vi "readShopInfo.vi"() -> (0 "数组 2":T1(array[cluster]))   [LabVIEW 2013, in "ShopBase.lvclass"]
uses:
  ShopBase.lvclass
  <vilib>/Utility/xml.llb/Read From XML File(string).vi
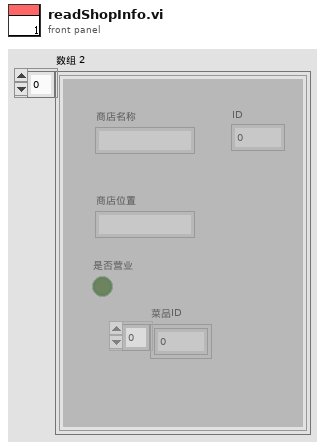
[diagram p1: front panel]
types:
  T1 = cluster{"ID":dbl, "商店名称":string, "商店位置":string, "是否营业":bool, "菜品ID":dbl[]}[]
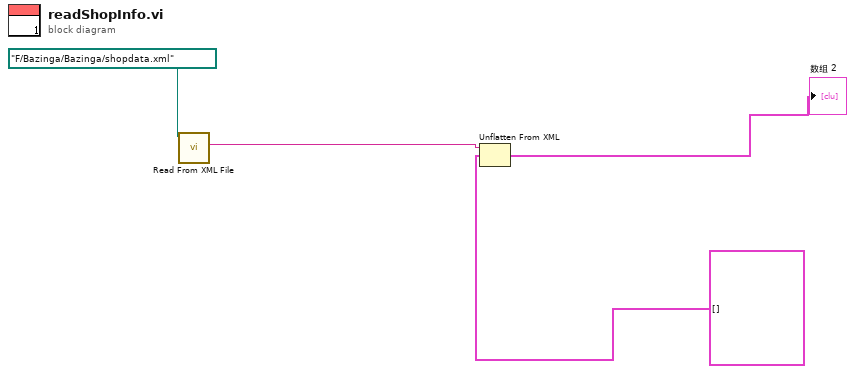
[diagram p0: block diagram]
diagram:
  n1 = call-poly <vilib>:"Read From XML File.vi"("XML File Path"=path "F:/Bazinga/Bazinga/shopdata.xml") -> ("XML Elements"=w3:string)  [unwired: 8 in, 2 out]
  n2 = Unflatten From XML(xml string=w3, type=T1 []) -> (value=→"数组 2":T1)  [unwired: 1 in, 1 out]
